vi "Predict GB Dimensions 2014-11-29.vi"(10 "Tolerance":dbl=0.001, 11 "Grain Boundary Macro Definition":T3={"Grain 1 Orientation"=[1.0, 0.6019417241891012, 0.029651947654046266], "Grain 2 Orientation"=[1.0, 0.730727623275494, 0.2205637301176], "Twist Angle (Deg)"=0.0}) -> (1 "Height Error":dbl, 2 "Width Error":dbl, 3 "Suggested Dimensions":T1)   [LabVIEW 2010]
uses:
  <vilib>/Analysis/Matrix/Datatypes/RealMatrix.ctl
  <vilib>/Analysis/baseanly.llb/Real A x B.vi
  <vilib>/Analysis/baseanly.llb/A x Vector.vi
  <vilib>/Analysis/NI_AALPro.lvlib
  <vilib>/Analysis/NI_AALBase.lvlib
  <vilib>/Analysis/Matrix/NI_Matrix.lvlib
panel:
  out "Suggested Dimensions 2":T1
  out "Grain 2 Height":dbl
  out "Grain 1 Height":dbl
  out "Grain 2 Width":dbl
  out "Grain 1 Width":dbl
  in  "Lattice Parameter":dbl=6.615785553057252
  out "Try this height":dbl
  out "Try this width":dbl
  out "Suggested X 2":dbl
  out "Suggested Y 2":dbl
  out "Suggested Grain 2 Length":dbl
  out "Suggested Grain 1 Length":dbl
  out "Suggested Y":dbl
  out "Suggested X":dbl
  out "Grain A":T2
  out "Grain B":T2
  out "Tilt Angle":dbl=10.024929742348679
  in  "Mutual Viewing Angle":dbl[](array[numeric])=[1.0, -1.6612903871170226, 0.0]
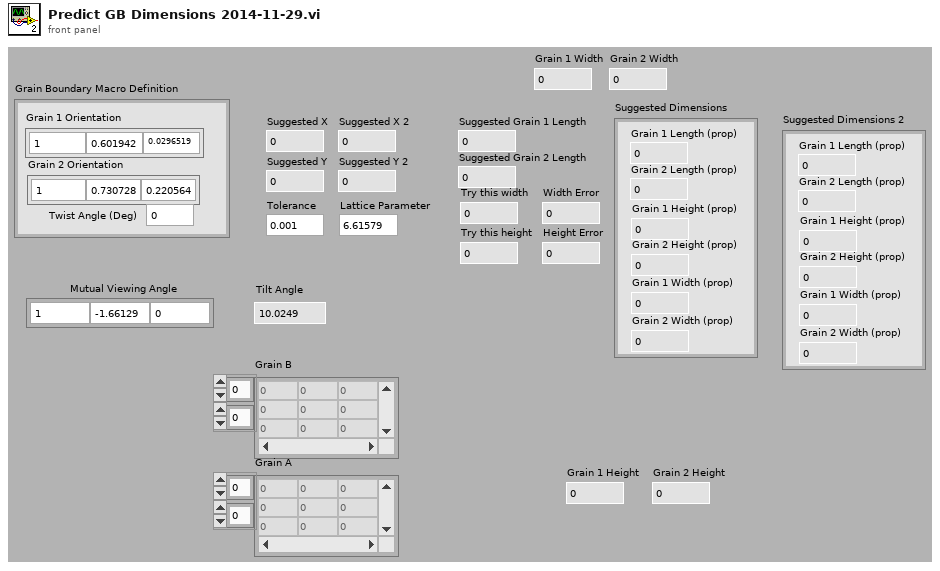
[diagram p1: front panel]
types:
  T1 = cluster{"Grain 1 Length (prop)":dbl, "Grain 2 Length (prop)":dbl, "Grain 1 Height (prop)":dbl, "Grain 2 Height (prop)":dbl, "Grain 1 Width (prop)":dbl, "Grain 2 Width (prop)":dbl}
  T2 = typedef "NI_Matrix.lvlib/RealMatrix.ctl" = dbl[][]
  T3 = cluster{"Grain 1 Orientation":dbl[], "Grain 2 Orientation":dbl[], "Twist Angle (Deg)":dbl}
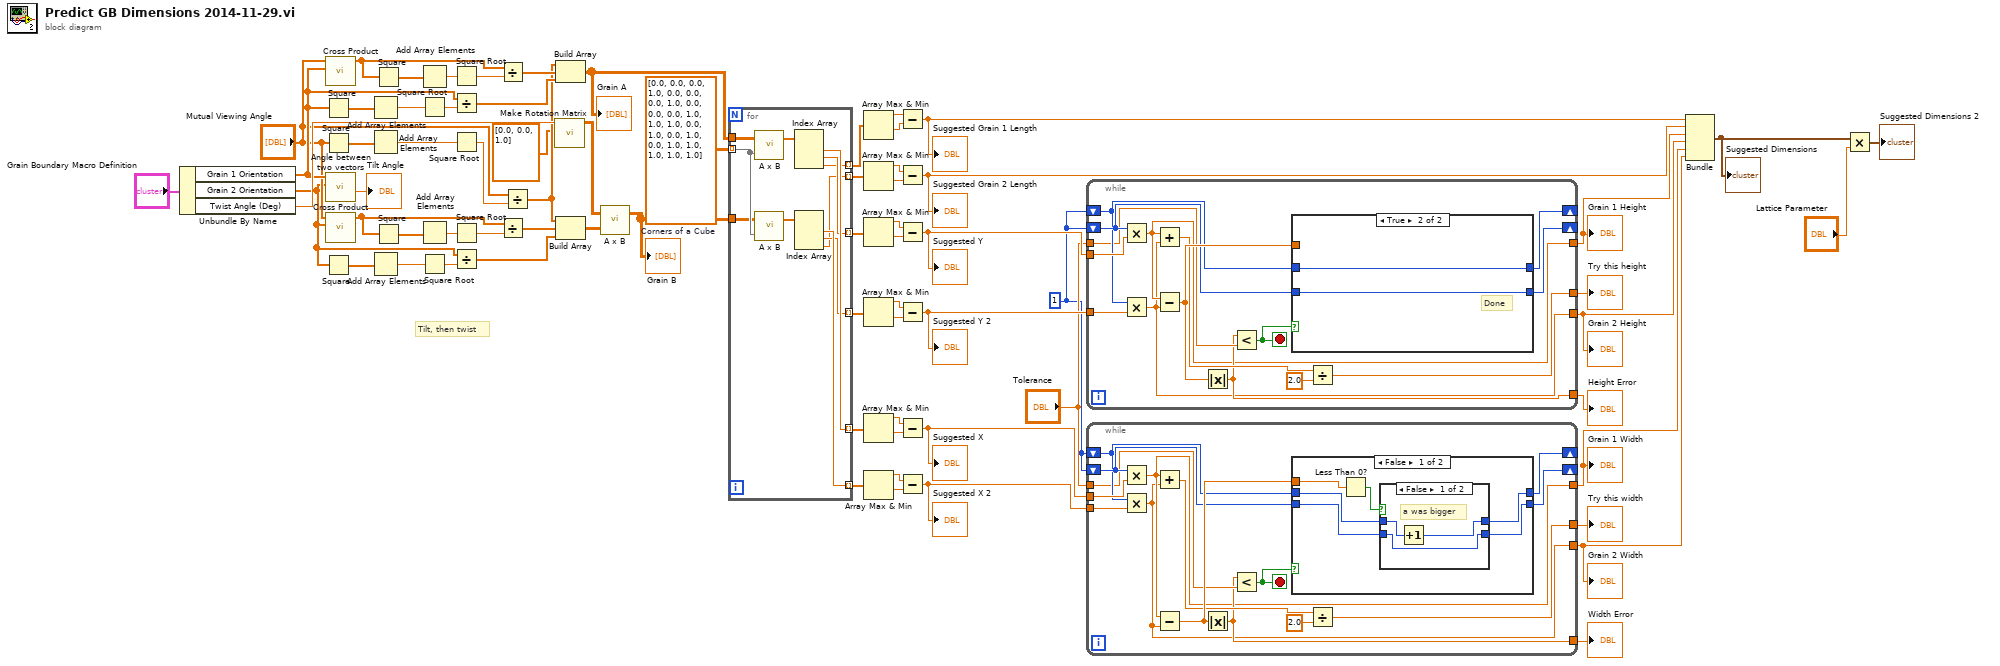
[diagram p0: block diagram]
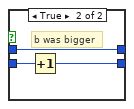
[diagram p2: hidden frame]
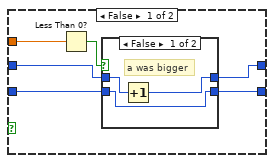
[diagram p4: hidden frame]
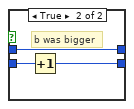
[diagram p5: hidden frame]
diagram:
  w62 = dbl[][] [[0.0, 0.0, 0.0], [1.0, 0.0, 0.0], [0.0, 1.0, 0.0], [0.0, 0.0, 1.0], [1.0, 1.0, 0.0], [1.0, 0.0, 1.0], [0.0, 1.0, 1.0], [1.0, 1.0, 1.0]]  # Corners of a Cube
  w36 = 1
  # "Tilt, then twist"
  n1 = Unbundle By Name("Grain Boundary Macro Definition") -> ("Grain 1 Orientation"=w22:dbl[], "Grain 2 Orientation"=w2:dbl[], "Twist Angle (Deg)"=w64:dbl)
  n2 = Square(x=w22) -> (x^2=w21:dbl[])
  n3 = Square(x="Mutual Viewing Angle") -> (x^2=w17:dbl[])
  n4 = Square(x=w2) -> (x^2=w3:dbl[])
  n5 = call <vilib>:"Cross Product.vi"("B Vector"=w22, "A Vector"="Mutual Viewing Angle") -> ("Cross Product"=w11:dbl[])  [unwired: 8 in, 1 out]
  n6 = call "Angle between two vectors.vi"("Vector 2"=w2, "Vector 1"=w22) -> ("Angle (Degrees)"=→"Tilt Angle":dbl)  [unwired: 7 in, 2 out]
  n7 = call <vilib>:"Cross Product.vi"("B Vector"=w2, "A Vector"="Mutual Viewing Angle") -> ("Cross Product"=w7:dbl[])  [unwired: 8 in, 1 out]
  n8 = Add Array Elements(numeric array=w21) -> (sum=w20:dbl)
  n9 = Add Array Elements(numeric array=w17) -> (sum=w18:dbl)
  n10 = Add Array Elements(numeric array=w3) -> (sum=w4:dbl)
  n11 = Square(x=w11) -> (x^2=w13:dbl[])
  n12 = Square(x=w7) -> (x^2=w9:dbl[])
  n13 = Add Array Elements(numeric array=w13) -> (sum=w12:dbl)
  n14 = Square Root(x=w20) -> (sqrt(x)=w19:dbl)
  n15 = Add Array Elements(numeric array=w9) -> (sum=w8:dbl)
  n16 = Square Root(x=w4) -> (sqrt(x)=w1:dbl)
  n17 = Square Root(x=w12) -> (sqrt(x)=w10:dbl)
  n18 = Divide(x=w22, y=w19) -> (x/y=w71:dbl[])
  n19 = Square Root(x=w18) -> (sqrt(x)=w14:dbl)
  n20 = Square Root(x=w8) -> (sqrt(x)=w6:dbl)
  n21 = Divide(x=w2, y=w1) -> (x/y=w67:dbl[])
  n22 = Divide(x=w11, y=w10) -> (x/y=w70:dbl[])
  n23 = Divide(x=w7, y=w6) -> (x/y=w69:dbl[])
  n24 = Divide(x="Mutual Viewing Angle", y=w14) -> (x/y=w16:dbl[])
  n25 = call "Make Rotation Matrix.vi"("Rotation Axis"=dbl[] [0.0, 0.0, 1.0], "Rotation Angle (Degree)"=w64) -> ("Rotation Matrix"=w68:T2)  [unwired: 9 in]
  n26 = Build Array(w16, w70, w71) -> (w61:T2)
  "Grain A" <- w61
  n27 = Build Array(w16, w69, w67) -> (w65:T2)
  n28 = call-poly <vilib>:"A x B.vi"("B"=w65, "A"=w68) -> ("A x B"=w60:T2)  [unwired: 1 out]
  "Grain B" <- w60
  n29 = for {
    tunnel: w62 -> [w81] mode=indexing
    tunnel: w61 -> [w82]
    tunnel: w60 -> [w80]
    tunnel: [w77] -> w53 mode=indexing
    tunnel: [w76] -> w52 mode=indexing
    tunnel: [w75] -> w51 mode=indexing
    tunnel: [w74] -> w44 mode=indexing
    tunnel: [w73] -> w43 mode=indexing
    tunnel: [w72] -> w42 mode=indexing
    n30 = call-poly <vilib>:"A x B.vi"("Vector"=w81, "A"=w82) -> ("A x Vector"=w79:dbl[])  [unwired: 1 out]
    n31 = call-poly <vilib>:"A x B.vi"("Vector"=w81, "A"=w80) -> ("A x Vector"=w78:dbl[])  [unwired: 1 out]
    n32 = Index Array(array=w79) -> (element #1=w77:dbl, element #2=w76:dbl, element #3=w75:dbl)  [unwired: 3 in]
    n33 = Index Array(array=w78) -> (element #1=w74:dbl, element #2=w73:dbl, element #3=w72:dbl)  [unwired: 3 in]
  }
  n34 = Array Max & Min(array=w51) -> (max value=w55:dbl, min value=w54:dbl)  [unwired: 2 out]
  n35 = Array Max & Min(array=w42) -> (max value=w49:dbl, min value=w50:dbl)  [unwired: 2 out]
  n36 = Array Max & Min(array=w52) -> (max value=w56:dbl, min value=w57:dbl)  [unwired: 2 out]
  n37 = Array Max & Min(array=w43) -> (max value=w48:dbl, min value=w47:dbl)  [unwired: 2 out]
  n38 = Array Max & Min(array=w53) -> (max value=w59:dbl, min value=w58:dbl)  [unwired: 2 out]
  n39 = Array Max & Min(array=w44) -> (max value=w45:dbl, min value=w46:dbl)  [unwired: 2 out]
  n40 = Subtract(x=w55, y=w54) -> (x-y=w34:dbl)
  "Suggested Grain 1 Length" <- w34
  n41 = Subtract(x=w49, y=w50) -> (x-y=w33:dbl)
  "Suggested Grain 2 Length" <- w33
  n42 = Subtract(x=w56, y=w57) -> (x-y=w41:dbl)
  "Suggested Y" <- w41
  n43 = Subtract(x=w48, y=w47) -> (x-y=w40:dbl)
  "Suggested Y 2" <- w40
  n44 = Subtract(x=w59, y=w58) -> (x-y=w38:dbl)
  "Suggested X" <- w38
  n45 = Subtract(x=w45, y=w46) -> (x-y=w37:dbl)
  "Suggested X 2" <- w37
  n46 = while {
    shift-right: [w92] -> _
    shift-left: w36 -> [w93]
    shift-right: [w90] -> _
    shift-left: w36 -> [w91]
    tunnel: w41 -> [w97]
    tunnel: w40 -> [w96]
    tunnel: [w86] -> w32
    tunnel: "Tolerance" -> [w89]
    tunnel: [w85] -> w35
    tunnel: [w84] -> w28
    tunnel: [w83] -> w27
    stop <- w95 stop-if-true
    n47 = Multiply(x=w93, y=w97) -> (x*y=w84:dbl)
    n48 = Multiply(x=w91, y=w96) -> (x*y=w83:dbl)
    n49 = Add(x=w84, y=w83) -> (x+y=w87:dbl)
    n50 = Subtract(x=w84, y=w83) -> (x-y=w94:dbl)
    n51 = Absolute Value(x=w94) -> (abs(x)=w85:dbl)
    n52 = Less?(x=w85, y=w89) -> (x < y?=w95:bool)
    n53 = case shown="True" w95 {
      tunnel: w94 -> [w103 _]
      tunnel: w93 -> [w102 w111]
      tunnel: [w101 w111] -> w92
      tunnel: w91 -> [w100 w110]
      tunnel: [w99 w110] -> w90
      frame False {
        n54 = Less Than 0?(x=w103) -> (x < 0?=w98:bool)
        n55 = case shown="False" w98 {
          tunnel: w102 -> [w104 w109]
          tunnel: [w104 w108] -> w101
          tunnel: w100 -> [w106 w107]
          tunnel: [w105 w107] -> w99
          frame False {
            # "a was bigger"
            n56 = Increment(x=w106) -> (x+1=w105:i32)
          }
          frame True {
            # "b was bigger"
            n57 = Increment(x=w109) -> (x+1=w108:i32)
          }
        }
      }
      frame True {
        # "Done"
      }
    }
    n58 = Divide(x=w87, y=2.0) -> (x/y=w86:dbl)
  }
  "Try this height" <- w32
  "Height Error" <- w35
  "Grain 1 Height" <- w28
  "Grain 2 Height" <- w27
  n59 = while {
    shift-right: [w121] -> _
    shift-left: w36 -> [w122]
    shift-right: [w119] -> _
    shift-left: w36 -> [w120]
    tunnel: w38 -> [w126]
    tunnel: w37 -> [w125]
    tunnel: [w115] -> w30
    tunnel: "Tolerance" -> [w118]
    tunnel: [w114] -> w31
    tunnel: [w113] -> w26
    tunnel: [w112] -> w25
    stop <- w124 stop-if-true
    n60 = Multiply(x=w122, y=w126) -> (x*y=w113:dbl)
    n61 = Multiply(x=w120, y=w125) -> (x*y=w112:dbl)
    n62 = Add(x=w113, y=w112) -> (x+y=w116:dbl)
    n63 = Subtract(x=w113, y=w112) -> (x-y=w123:dbl)
    n64 = Absolute Value(x=w123) -> (abs(x)=w114:dbl)
    n65 = Less?(x=w114, y=w118) -> (x < y?=w124:bool)
    n66 = case shown="False" w124 {
      tunnel: w123 -> [w132 _]
      tunnel: w122 -> [w131 w140]
      tunnel: [w130 w140] -> w121
      tunnel: w120 -> [w129 w139]
      tunnel: [w128 w139] -> w119
      frame False {
        n67 = Less Than 0?(x=w132) -> (x < 0?=w127:bool)
        n68 = case shown="False" w127 {
          tunnel: w131 -> [w133 w138]
          tunnel: [w133 w137] -> w130
          tunnel: w129 -> [w135 w136]
          tunnel: [w134 w136] -> w128
          frame False {
            # "a was bigger"
            n69 = Increment(x=w135) -> (x+1=w134:i32)
          }
          frame True {
            # "b was bigger"
            n70 = Increment(x=w138) -> (x+1=w137:i32)
          }
        }
      }
      frame True {
        # "Done"
      }
    }
    n71 = Divide(x=w116, y=2.0) -> (x/y=w115:dbl)
  }
  "Try this width" <- w30
  "Width Error" <- w31
  "Grain 1 Width" <- w26
  "Grain 2 Width" <- w25
  n72 = Bundle(w34, w33, w28, w27, w26, w25) -> (w24:cluster{dbl, dbl, dbl, dbl, dbl, dbl})  [unwired: 1 in]
  "Suggested Dimensions" <- w24
  n73 = Multiply(x=w24, y="Lattice Parameter") -> (x*y=→"Suggested Dimensions 2":cluster{dbl, dbl, dbl, dbl, dbl, dbl})
